vi "Pointcloud Create.vi"(8 "error in (no error)":errorcluster, 9 "Width":i32, 10 "Height":i32, 11 "Pointcloud in":refnum<class "Pointcloud.lvclass">) -> (0 "error out":errorcluster, 3 "Pointcloud out":refnum<class "Pointcloud.lvclass">)   [LabVIEW 2018, in "Pointcloud.lvclass"]
uses:
  Pointcloud.lvclass
  <vilib>/Utility/miscctls.llb/LV3DPointTypeDef.ctl
  <vilib>/Utility/miscctls.llb/LVRGBAColorTypeDef.ctl
  Pointcloud.lvclass/Pointcloud.ctl
  <vilib>/picture/3D Picture Control/NI_3D Picture Control.lvlib
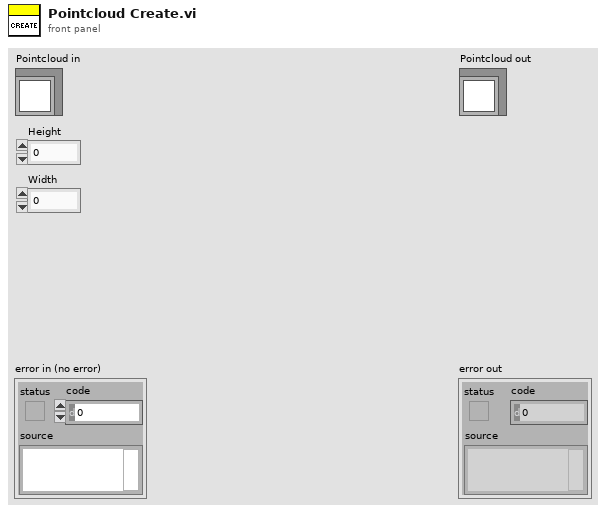
[diagram p1: front panel]
types:
  T1 = typedef "LVRGBAColorTypeDef.ctl" = cluster{"Red":sgl, "Green":sgl, "Blue":sgl, "Alpha":sgl}
  T2 = typedef "LV3DPointTypeDef.ctl" = cluster{"X":sgl, "Y":sgl, "Z":sgl}
  T3 = cluster{"Alpha":sgl, "Blue":sgl, "Green":sgl, "Red":sgl}
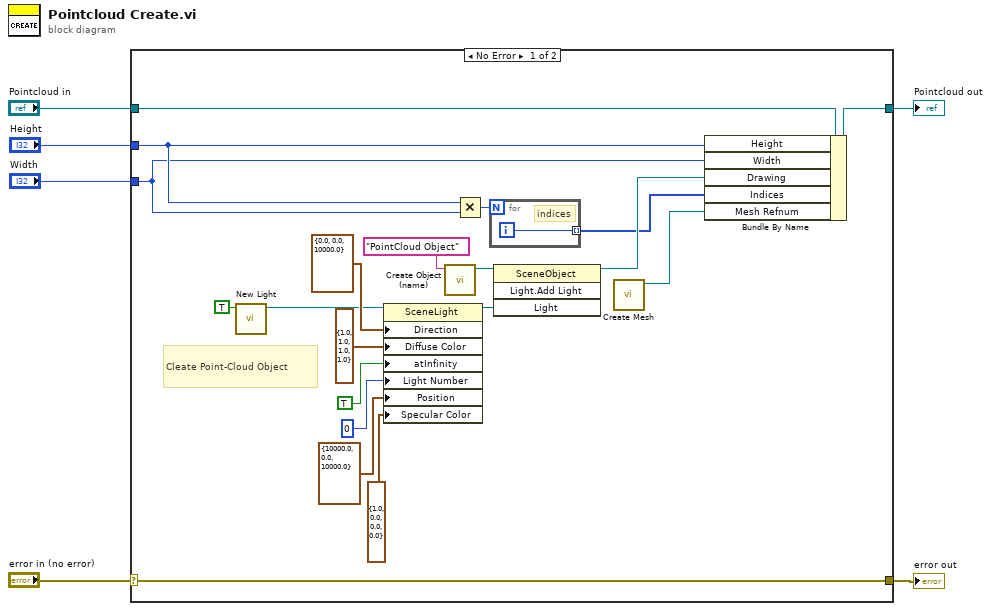
[diagram p0: block diagram]
diagram:
  n1 = case shown="No Error" "error in (no error)" {
    selector: "error in (no error)" -> [w26 w29]
    tunnel: [w26 w29] -> w5
    tunnel: [w24 w28] -> w3
    tunnel: "Pointcloud in" -> [w25 w28]
    tunnel: "Height" -> [w8 _]
    tunnel: "Width" -> [w7 _]
    frame No Error {
      # "Cleate Point-Cloud Object"
      n2 = call <vilib>:"New Light.vi"("At Infinity"=TRUE) -> ("New Light Refnum"=w17:refnum<vi>)  [unwired: 2 in, 8 out]
      n3 = property class="SceneLight"(reference=w17, "Direction"=cluster{"X":sgl, "Y":sgl, "Z":sgl} {"X"=0.0, "Y"=0.0, "Z"=10000.0}, "Diffuse Color"=T3 {"Alpha"=1.0, "Blue"=1.0, "Green"=1.0, "Red"=1.0}, "atInfinity"=TRUE ("At Infinity"), "Light Number"=0, "Position"=T2 {"X"=10000.0, "Y"=0.0, "Z"=10000.0}, "Specular Color"=T1 {"Red"=1.0, "Green"=0.0, "Blue"=0.0, "Alpha"=0.0}) -> (reference out=w14:refnum<vi>)  [unwired: 1 in, 1 out]
      n4 = call <vilib>:"Create Object (name).vi"("Name"="PointCloud Object") -> ("Scene:New Object"=w16:refnum<vi>)  [unwired: 9 in, 1 out]
      n5 = Multiply(x=w8, y=w7) -> (x*y=w9:i32)
      n6 = for {
        N: w9 -> [_]
        tunnel: [w27] -> w22 mode=indexing
        i -> [w27]
        # "indices"
      }
      n7 = invoke class="SceneObject" method="Light.Add Light"(reference=w16, "Light"=w14) -> (reference out=w23:refnum<vi>)  [unwired: 2 in, 3 out]
      n8 = call <vilib>:"Create Mesh.vi"() -> ("New Mesh Refnum"=w21:refnum<vi>)  [unwired: 10 in, 1 out]
      n9 = Bundle By Name(cluster=w25, "Height"=w8, "Width"=w7, "Drawing"=w23, "Indices"=w22, "Mesh Refnum"=w21) -> (w24:refnum<class "Pointcloud.lvclass">)
    }
    frame Error {
    }
  }
  "error out" <- w5
  "Pointcloud out" <- w3
